vi "Process Data Message.vi"(8 "message data":variant, 10 "message":string, 11 "message type":string) -> ()   [LabVIEW 2016]
panel:
  in  "error in (no error)":errorcluster
  out "error out":errorcluster
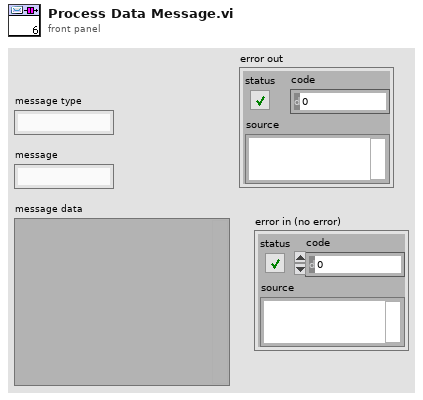
[diagram p1: front panel]
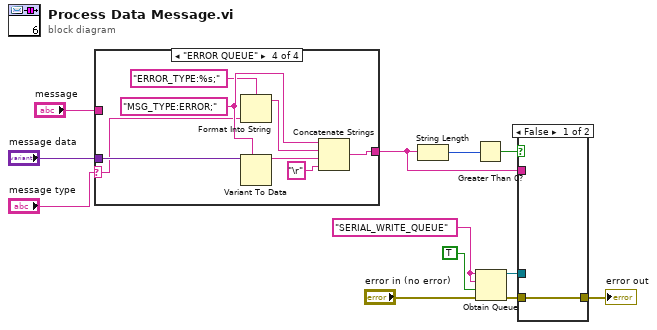
[diagram p0: block diagram]
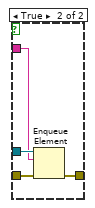
[diagram p2: hidden frame]
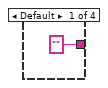
[diagram p3: hidden frame]
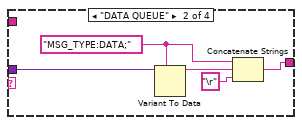
[diagram p4: hidden frame]
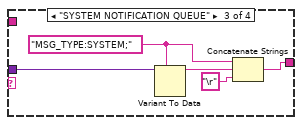
[diagram p5: hidden frame]
diagram:
  w7 = "SERIAL_WRITE_QUEUE"
  n1 = case shown="\"ERROR QUEUE\"" "message type" {
    selector: "message type" -> [_ _ _ w26]
    tunnel: "message data" -> [_ w16 w23 w29]
    tunnel: ["" w14 w19 w28] -> w3
    tunnel: "message" -> [_ _ _ _]
    frame Default {
    }
    frame "DATA QUEUE" {
      w15 = "MSG_TYPE:DATA;"
      n2 = Variant To Data(type=w15, Variant=w16) -> (data=w18:string)  [unwired: 1 in, 1 out]
      n3 = Concatenate Strings(w15, w18, "\r" ("string")) -> (w14:string)
    }
    frame "SYSTEM NOTIFICATION QUEUE" {
      w22 = "MSG_TYPE:SYSTEM;"
      n4 = Variant To Data(type=w22, Variant=w23) -> (data=w21:string)  [unwired: 1 in, 1 out]
      n5 = Concatenate Strings(w22, w21, "\r" ("string")) -> (w19:string)
    }
    frame "ERROR QUEUE" {
      w27 = "MSG_TYPE:ERROR;"
      n6 = Format Into String(format string="ERROR_TYPE:%s;", w26) -> (resulting string=w24:string)  [unwired: 2 in, 1 out]
      n7 = Variant To Data(type=w27, Variant=w29) -> (data=w31:string)  [unwired: 1 in, 1 out]
      n8 = Concatenate Strings(w27, w24, w31, "\r" ("string")) -> (w28:string)
    }
  }
  n9 = String Length(string=w3) -> (length=w9:i32)
  n10 = Greater Than 0?(x=w9) -> (x > 0?=w8:bool)
  n11 = Obtain Queue(name (unnamed)=w7, element data type=w7, create if not found? (T)=TRUE, error in (no error)="error in (no error)") -> (queue out=w5:refnum<queue>, error out=w4:errorcluster)  [unwired: 1 in, 1 out]
  n12 = case shown="False" w8 {
    tunnel: w5 -> [_ w36]
    tunnel: w4 -> [w32 w34]
    tunnel: w3 -> [_ w35]
    tunnel: [w32 w33] -> w2
    frame False {
    }
    frame True {
      n13 = Enqueue Element(queue=w36, element=w35, error in (no error)=w34) -> (error out=w33:errorcluster)  [unwired: 1 in, 2 out]
    }
  }
  "error out" <- w2
